vi "RS-xxx to GPIB ConvBox Factory Wrapper.vi"(8 "Error In":errorcluster, 10 "RS-xxx to GPIB ConvBox Settings":T1) -> (0 "Error Out":errorcluster, 3 "RS-xxx to GPIB ConvBox Out":refnum<class "RS-xxx to GPIB ConvBox.lvclass">)   [LabVIEW 2018, in "Instrument Addon Scripting API.lvlib"]
uses:
  Instrument Addon Scripting API.lvlib
  Addon/Support Libraries/Protocols.lvlibp/RS-xxx to GPIB ConvBox/RS-xxx to GPIB ConvBox Settings.ctl
  Addon/Support Libraries/Protocols.lvlibp/RS-xxx to GPIB ConvBox/RS-xxx to GPIB ConvBox.lvclass
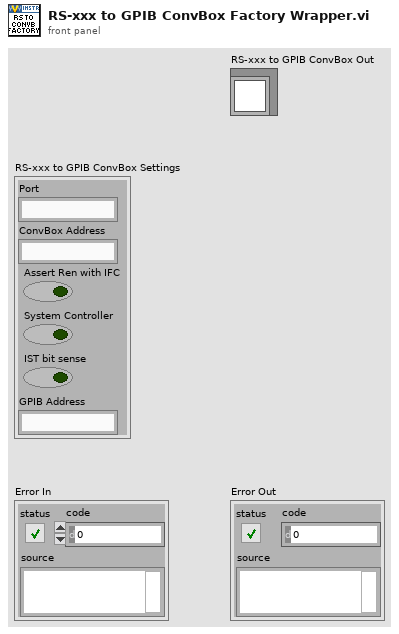
[diagram p1: front panel]
types:
  T1 = typedef "Protocols.lvlibp/RS-xxx to GPIB ConvBox.lvclass/RS-xxx to GPIB ConvBox Settings.ctl" = cluster{"Port":string, "ConvBox Address":string, "Assert Ren with IFC":bool, "System Controller":bool, "IST bit sense":bool, "GPIB Address":string}
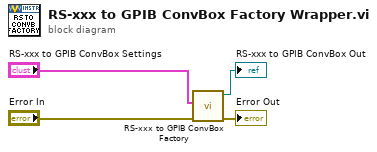
[diagram p0: block diagram]
diagram:
  n1 = call "RS-xxx to GPIB ConvBox Factory.vi"("Error In"="Error In", "RS-xxx to GPIB ConvBox Settings"="RS-xxx to GPIB ConvBox Settings") -> ("Error Out"=→"Error Out":errorcluster, "RS-xxx to GPIB ConvBox Out"=→"RS-xxx to GPIB ConvBox Out":refnum<class "RS-xxx to GPIB ConvBox.lvclass">)  [unwired: 8 in]
